vi "Calculate Response.vi"(0 "Neural Network In":refnum<class "Neural Network.lvclass">, 7 "Inputs":dbl[](array[numeric]), 11 "Error In":errorcluster) -> (4 "Neural Network Out":refnum<class "Neural Network.lvclass">, 8 "Outputs":dbl[](array[numeric]), 15 "Error Out":errorcluster)   [LabVIEW 2015, in "Neural Network.lvclass"]
doc: "Calculate the output values of the network based on the input values. \n\nThis VI also uses the scaling information generated by the teaching algorithm to scale the inputs and outputs of the network. This means that you can work with any values as long as you have tought the network in that specific range."
uses:
  Neural Network.lvclass
  <vilib>/Analysis/NI_AALBase.lvlib
  <vilib>/Analysis/baseanly.llb/A x Vector.vi
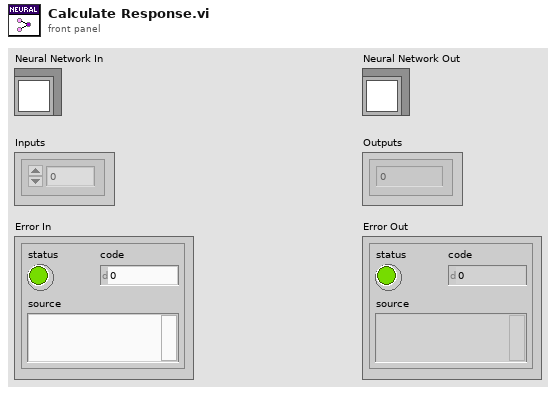
[diagram p1: front panel]
types:
  T1 = typedef "Neural Network.lvclass/Scaling Info.ctl" = cluster{"X Scaling Vector":dbl[], "Y Scaling Vector":dbl[]}
  T2 = typedef "Neural Network.lvclass/2D Array.ctl" = cluster{"2D Array":sgl[][]}
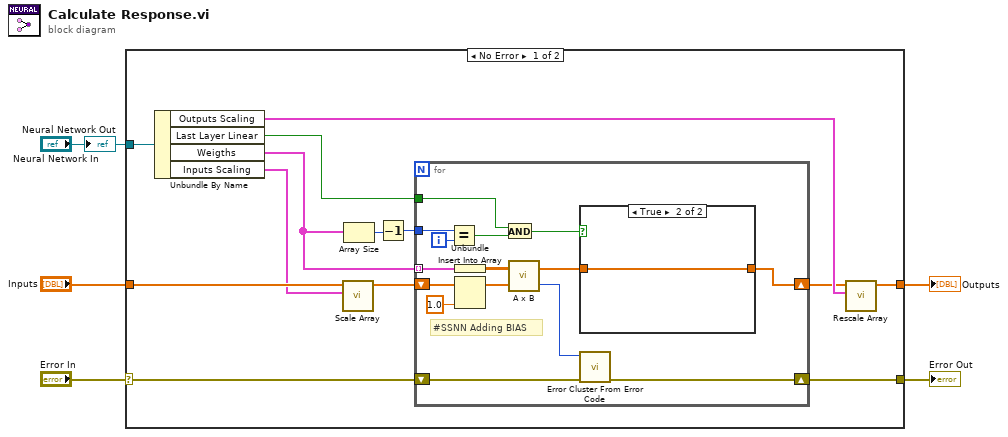
[diagram p0: block diagram]
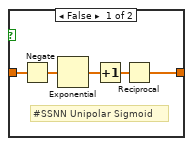
[diagram p2: hidden frame]
diagram:
  n1 = case shown="No Error" "Error In" {
    selector: "Error In" -> [w7 w40]
    tunnel: "Neural Network In" -> [w18 _]
    tunnel: "Inputs" -> [w15 _]
    tunnel: [w17 w40] -> w2
    tunnel: [w13 _] -> w1
    frame No Error {
      n2 = Unbundle By Name(w18) -> ("Outputs Scaling"=w12:T1, "Last Layer Linear"=w16:bool, "Weigths"=w8:T2[], "Inputs Scaling"=w14:T1)
      n3 = call "Scale Array.vi"("Scaling Info"=w14, "Array to Scale"=w15) -> ("Scaled Array"=w9:dbl[])  [unwired: 9 in]
      n4 = Array Size(array=w8) -> (size(s)=w11:i32)
      n5 = Decrement(x=w11) -> (x-1=w10:i32)
      n6 = for {
        shift-right: [w31] -> w6
        shift-left: w9 -> [w30]
        tunnel: w8 -> [w33] mode=indexing
        tunnel: w10 -> [w27]
        shift-right: [w20] -> w17
        shift-left: w7 -> [w21]
        tunnel: w16 -> [w22]
        i -> [w25]
        # "#SSNN Adding BIAS"
        n7 = Equal?(x=w27, y=w25) -> (x = y?=w26:bool)
        n8 = Unbundle(w33) -> ("2D Array"=w32:sgl[][])
        n9 = Insert Into Array(array=w30, new element=1.0 ("new element/subarray")) -> (w29:dbl[])  [unwired: 1 in]
        n10 = And(x=w22, y=w26) -> (x .and. y?=w23:bool)
        n11 = call-poly <vilib>:"A x B.vi"("Vector"=w29, "A"=w32) -> ("error"=w24:i32, "A x Vector"=w28:dbl[])
        n12 = case shown="True" w23 {
          tunnel: [w35 w39] -> w31
          tunnel: w28 -> [w34 w39]
          frame False {
            # "#SSNN Unipolar Sigmoid"
            n13 = Negate(x=w34) -> (-x=w38:dbl[])
            n14 = Exponential(1:w38) -> (0:w37:dbl[])
            n15 = Increment(x=w37) -> (x+1=w36:dbl[])
            n16 = Reciprocal(x=w36) -> (1/x=w35:dbl[])
          }
          frame True {
          }
        }
        n17 = call <vilib>:"Error Cluster From Error Code.vi"("error in (no error)"=w21, "error code (0)"=w24) -> ("error out"=w20:errorcluster)  [unwired: 7 in]
      }
      n18 = call "Rescale Array.vi"("Scaling Info"=w12, "Array to Rescale"=w6) -> ("Rescaled Array"=w13:dbl[])  [unwired: 9 in]
    }
    frame Error {
    }
  }
  "Error Out" <- w2
  "Outputs" <- w1
  "Neural Network Out" <- "Neural Network In"
